vi "pr_mod_v1.vi"() -> ()   [LabVIEW 2009]
panel:
  out "Presiunea":dbl(knob)=6.256275754376487 scale=0.0..10.0
  in  "stop":bool
  in  "Presiune maxima (bar)":dbl(slide)=6.7 scale=0.0..10.0
  out "Temperatura":dbl(slide)=16.387345825316686 scale=0.0..100.0
  in  "Temperatura maxima":dbl(slide)=64.0 scale=0.0..100.0
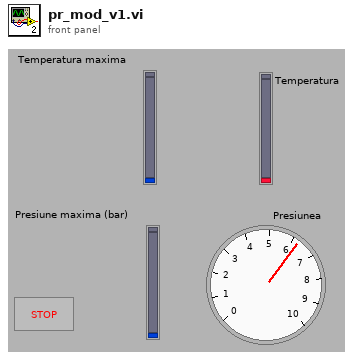
[diagram p1: front panel]
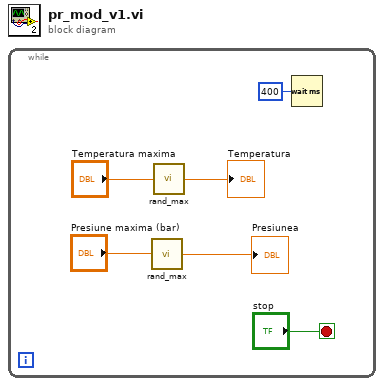
[diagram p0: block diagram]
diagram:
  n1 = while {
    stop <- "stop" stop-if-true
    n2 = call "rand_max.vi"("Val_max"="Presiune maxima (bar)") -> ("Val_out"=→"Presiunea":dbl)
    n3 = call "rand_max.vi"("Val_max"="Temperatura maxima") -> ("Val_out"=→"Temperatura":dbl)
    n4 = Wait (ms)(milliseconds to wait=u32 400) -> ()  [unwired: 1 out]
  }
